vi "DFConfig Get XPointers.vi"(11 "String":string) -> (3 "Xpointers":string[](array[string]))   [LabVIEW 2011]
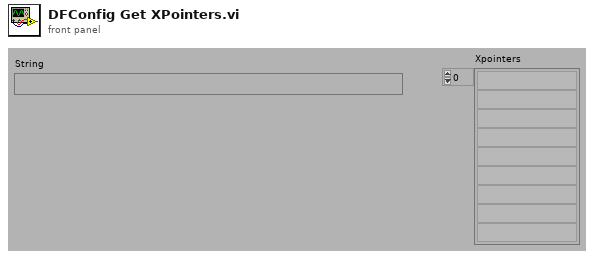
[diagram p1: front panel]
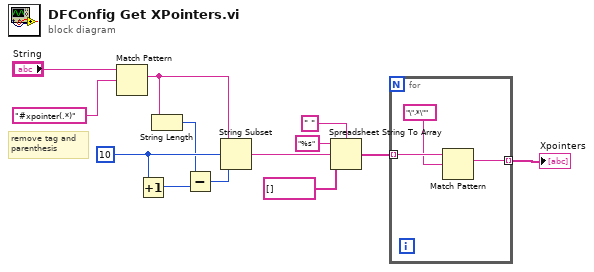
[diagram p0: block diagram]
diagram:
  w11 = 10 ("offset (0)")
  # "remove tag and\nparenthesis"
  n1 = Match Pattern(string="String", regular expression="#xpointer(.*)") -> (match substring=w8:string)  [unwired: 4 out]
  n2 = Increment(x=w11) -> (x+1=w10:i32)
  n3 = String Length(string=w8) -> (length=w9:i32)
  n4 = Subtract(x=w9, y=w10) -> (x-y=w7:i32)
  n5 = String Subset(string=w8, offset (0)=w11, length (rest)=w7) -> (substring=w3:string)
  n6 = Spreadsheet String To Array(delimiter (Tab)=" ", format string="%s", spreadsheet string=w3, array type (2D Dbl)=string[] [] ("Xpointers")) -> (array=w2:string[])
  n7 = for {
    tunnel: w2 -> [w16] mode=indexing
    tunnel: [w14] -> w1 mode=indexing
    n8 = Match Pattern(string=w16, regular expression="\".*\"" ("delimiter (Tab)")) -> (match substring=w14:string)  [unwired: 4 out]
  }
  "Xpointers" <- w1
